vi "TST.vi"(8 "error in":errorcluster, 11 "SCPI in":refnum<class "SCPI.lvclass">) -> (0 "error out":errorcluster, 2 "read buffer":string, 3 "SCPI out":refnum<class "SCPI.lvclass">)   [LabVIEW 2011, in "SCPI.lvclass"]
doc: "Run a self test."
uses:
  SCPI.lvclass
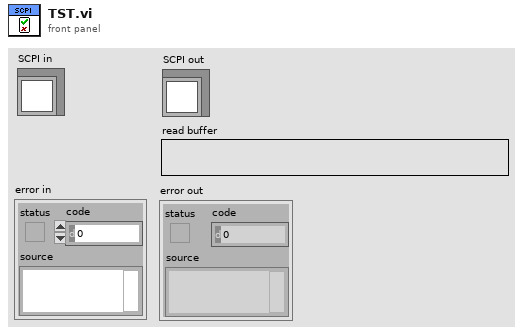
[diagram p1: front panel]
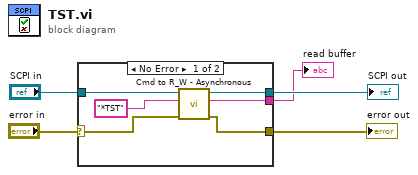
[diagram p0: block diagram]
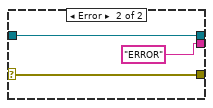
[diagram p2: hidden frame]
diagram:
  n1 = case shown="No Error" "error in" {
    selector: "error in" -> [w8 w14]
    tunnel: [w7 w14] -> w4
    tunnel: [w10 w13] -> w2
    tunnel: "SCPI in" -> [w11 w13]
    tunnel: [w6 "ERROR" ("read buffer")] -> w1
    frame No Error {
      n2 = call-dynamic "Cmd to R_W - Asynchronous.vi"("error in"=w8, "write buffer"="*TST", "Serial IO in"=w11) -> ("error out"=w7:errorcluster, "read buffer"=w6:string, "Serial IO out"=w10:refnum<class "SCPI.lvclass">)  [unwired: 6 in]
    }
    frame Error {
    }
  }
  "error out" <- w4
  "SCPI out" <- w2
  "read buffer" <- w1
